vi "save_log_02.vi"() -> ()   [LabVIEW 2024]
panel:
  in  "错误输入":errorcluster
  out "错误输出":errorcluster
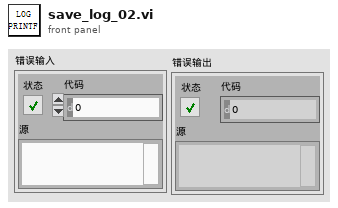
[diagram p1: front panel]
types:
  T1 = enum16{"open", "replace", "create", "open or create", "replace or create", "replace or create with confirmation"}
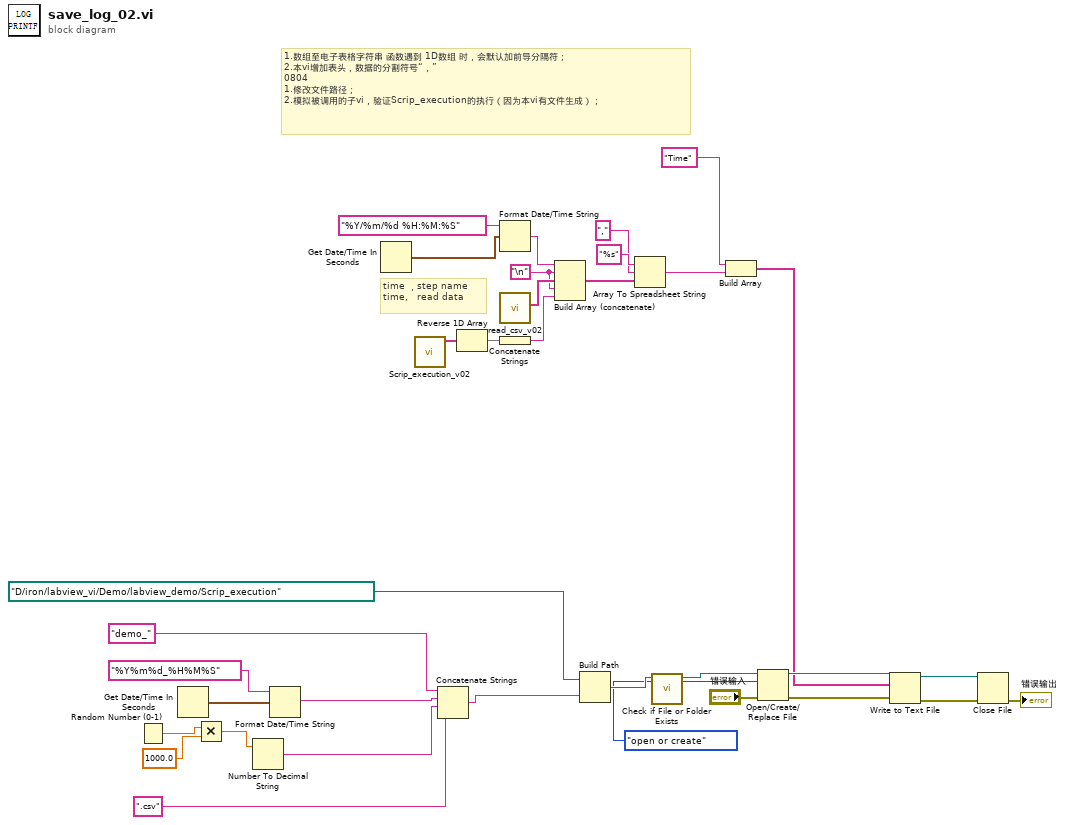
[diagram p0: block diagram]
diagram:
  w5 = "\n"
  # "time ，step name\ntime,   read data"
  # "1.数组至电子表格字符串 函数遇到 1D数组 时，会默认加前导分隔符；\n2.本vi增加表头，数据的分割符号“，”\n0804\n1.修改文件路径；\n2.模拟被调用的子vi，验证Scrip_execution的执行（因为本vi有文件生成）；"
  n1 = Random Number (0-1)() -> (number: 0 to 1=w13:dbl)
  n2 = Get Date/Time In Seconds() -> (seconds since 1Jan1904=w22:timestamp)
  n3 = Multiply(x=w13, y=1000.0) -> (x*y=w11:dbl)
  n4 = Number To Decimal String(number=w11) -> (decimal integer string=w10:string)  [unwired: 1 in]
  n5 = Format Date/Time String(time format string (%c)="%Y%m%d_%H%M%S" ("时间格式字符串(%c)"), seconds (now)=w22) -> (date/time string=w21:string)  [unwired: 1 in]
  n6 = Get Date/Time In Seconds() -> (seconds since 1Jan1904=w32:timestamp)
  n7 = call "Scrip_execution_v02.vi"() -> ("添加的数组"=w2:string[])  [unwired: 11 in]
  n8 = Concatenate Strings("demo_" ("字符串"), w21, w10, ".csv" ("字符串")) -> (w24:string)
  n9 = Reverse 1D Array(array=w2) -> (reversed array=w1:string[])
  n10 = Format Date/Time String(time format string (%c)="%Y/%m/%d %H:%M:%S" ("时间格式字符串(%c)"), seconds (now)=w32) -> (date/time string=w6:string)  [unwired: 1 in]
  n11 = call "read_csv_v02.vi"() -> ("Step name 给log表头"=w8:string[])  [unwired: 10 in, 1 out]
  n12 = Concatenate Strings(w1) -> (w3:string)
  n13 = Build Array (concatenate)(w6, w5, w8, w5, w3) -> (w30:string[])
  n14 = Build Path(base path=path "D:/iron/labview_vi/Demo/labview_demo/Scrip_execution" ("基路径"), name or relative path=w24) -> (appended path=w34:path)
  n15 = Array To Spreadsheet String(delimiter (Tab)="," ("分隔符(Tab)"), array=w30, 3:"%s" ("格式字符串")) -> (spreadsheet string=w19:string)
  n16 = call <vilib>:"Check if File or Folder Exists.vi"("path"=w34) -> ("dup path"=w33:path)  [unwired: 8 in, 2 out]
  n17 = Build Array("Time" ("元素"), w19) -> (w18:string[])
  n18 = Open/Create/Replace File(file path (use dialog)=w33, error in="错误输入", operation (0:open)=T1."open or create" ("操作(0:open)")) -> (refnum out=w28:refnum<file>, error out=w17:errorcluster)  [unwired: 3 in, 1 out]
  n19 = Write to Text File(file (use dialog)=w28, text=w18, error in=w17) -> (refnum out=w27:refnum<file>, error out=w16:errorcluster)  [unwired: 1 in, 1 out]
  n20 = Close File(refnum=w27, error in=w16) -> (error out=→"错误输出":errorcluster)  [unwired: 1 out]
